vi "WPI_MotorControlClose.vi"(8 "error in (no error)":errorcluster, 11 "MotorControlDevRef":T1={"DeviceStatus"={"status"=FALSE, "code"=0, "source"=""}, "Type"=enum."PWM", "PWM"={"PWM Channel"=enum."PWM 1", "DeadBand"={"Name"="", "maxPositivePwm"=0, "minPositivePwm"=0, "centerPwm"=0, "maxNegativePwm"=0, "minNegativePwm"=0, "angularRange"=0}}, "CAN"={"Device Number"=0, "SetOutput VI Ref"=variant(enum8{"Percent VBus", "Current", "Speed", "Position", "Voltage"} enum."Percent VBus"), "GetOutput VI Ref"=variant(refnum<k1> refnum), "Enable VI Ref"=variant(dbl 12.0), "Disable VI Ref"=variant(enum8{"Percent VBus", "Speed", "Position", "Slave", "Unchanged / Invalid"} enum."Percent VBus"), "Data"=variant}, "Invert"=FALSE, "DIO PWM"={"PWM \"Enable\" Channel"=enum."Invalid", "DIOChannel"=enum."Invalid", "PWM Rate"=0.0}}) -> (0 "error out":errorcluster)   [LabVIEW 2017]
doc: "Closes the reference to the motor controller you specify. Use this VI to close each motor control reference that you open with the Open VI.\n\nThis software is licensed. Open the labview\\readme\\WPI Robotics Library Open Source License.txt file for more information."
uses:
  <vilib>/Rock Robotics/WPI/MotorControl/WPI_MotorControlDeviceRef.ctl
  <vilib>/Rock Robotics/WPI/MotorControl/WPI_MotorControlType.ctl
  <vilib>/Rock Robotics/SystemInterfaces/DIO/FPGA_DIOPWMChannel.ctl
  <vilib>/Rock Robotics/WPI/PWM/WPI_PWMDeadband.ctl
  <vilib>/Rock Robotics/SystemInterfaces/DIO/FPGA_DIOChannel.ctl
  <vilib>/Rock Robotics/WPI/PWM/WPI_PWMChannelCacheOp.ctl
  <instrlib>/DC Motor Controller/HAIOL/DC Motor Controller.lvclass
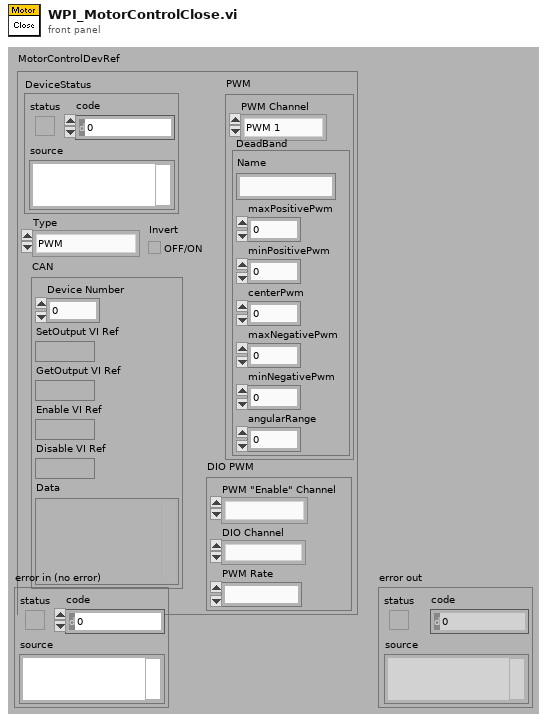
[diagram p1: front panel]
types:
  T1 = typedef "WPI_MotorControlDeviceRef.ctl" = cluster{"DeviceStatus":errorcluster, "Type":T2, "PWM":cluster{"PWM Channel":T3, "DeadBand":T4}, "CAN":cluster{"Device Number":u8, "SetOutput VI Ref":variant, "GetOutput VI Ref":variant, "Enable VI Ref":variant, "Disable VI Ref":variant, "Data":variant}, "Invert":bool, "DIO PWM":cluster{"PWM \"Enable\" Channel":T3, "DIOChannel":T5, "PWM Rate":dbl}}
  T2 = typedef "WPI_MotorControlType.ctl" = enum16{"PWM", "CAN", "DIO PWM"}
  T3 = typedef "FPGA_DIOPWMChannel.ctl" = enum8{"PWM 0", "PWM 1", "PWM 2", "PWM 3", "PWM 4", "PWM 5", "PWM 6", "PWM 7", "PWM 8", "PWM 9", "PWM MXP 0", "PWM MXP 1", "PWM MXP 2", "PWM MXP 3", "PWM MXP 4", "PWM MXP 5", "PWM MXP 6", "PWM MXP 7", "PWM MXP 8", "PWM MXP 9", "Invalid"}
  T4 = typedef "WPI_PWMDeadband.ctl" = cluster{"Name":string, "maxPositivePwm":i32, "minPositivePwm":i32, "centerPwm":i32, "maxNegativePwm":i32, "minNegativePwm":i32, "angularRange":u16}
  T5 = typedef "FPGA_DIOChannel.ctl" = enum8{"DIO 0", "DIO 1", "DIO 2", "DIO 3", "DIO 4", "DIO 5", "DIO 6", "DIO 7", "DIO 8", "DIO 9", "DIO MXP 0", "DIO MXP 1", "DIO MXP 2", "DIO MXP 3", "DIO MXP 4", "DIO MXP 5", "DIO MXP 6", "DIO MXP 7", "DIO MXP 8", "DIO MXP 9", "DIO MXP 10", "DIO MXP 11", "DIO MXP 12", "DIO MXP 13", "DIO MXP 14", "DIO MXP 15", "SPI Port CS1", "SPI Port CS2", "SPI Port CS3", "SPI Port MISO", "SPI Port MOSI", "Invalid"}
  T6 = typedef "WPI_PWMChannelCacheOp.ctl" = enum16{"Acquire", "Release", "Status"}
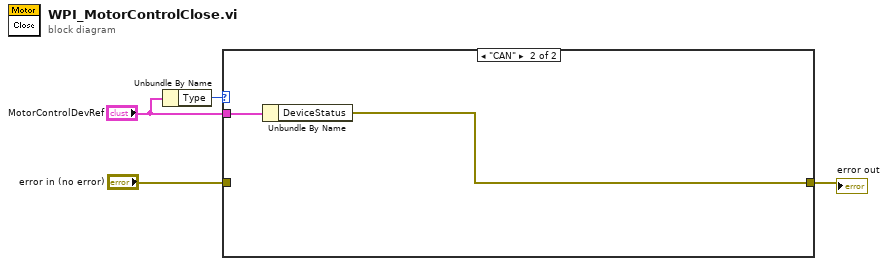
[diagram p0: block diagram]
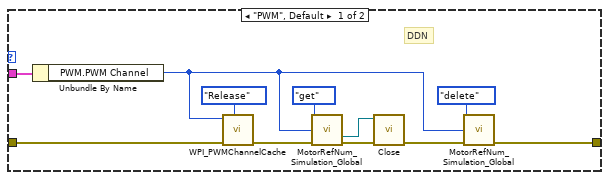
[diagram p2: hidden frame]
diagram:
  n1 = Unbundle By Name("MotorControlDevRef") -> ("Type"=w1:T2)
  n2 = case shown="\"CAN\"" w1 {
    tunnel: "error in (no error)" -> [w7 _]
    tunnel: [w6 w16] -> w3
    tunnel: "MotorControlDevRef" -> [w15 w17]
    frame "PWM", Default {
      # "DDN"
      n3 = Unbundle By Name(w15) -> ("PWM.PWM Channel"=w8:T3)
      n4 = call <vilib>:"WPI_PWMChannelCache.vi"("Operation"=WPI_PWMChannelCacheOp."Release", "error in (no error)"=w7, "PWMChannel"=w8) -> ("error out"=w12:errorcluster)  [unwired: 2 in, 6 out]
      n5 = call <vilib>:"MotorRefNum_Simulation_Global.vi"("menu"=enum16{"set", "get", "delete"}."get", "PWM Channel"=w8, "error in (no error)"=w12) -> ("DC Motor Controller Get"=w5:refnum<class "DC Motor Controller.lvclass">, "error out"=w11:errorcluster)  [unwired: 11 in]
      n6 = call-dynamic "Close.vi"("error in (no error)"=w11, "DC Motor Controller in"=w5) -> ("error out"=w9:errorcluster)  [unwired: 9 in]
      n7 = call <vilib>:"MotorRefNum_Simulation_Global.vi"("menu"=enum16{"set", "get", "delete"}."delete", "PWM Channel"=w8, "error in (no error)"=w9) -> ("error out"=w6:errorcluster)  [unwired: 11 in, 1 out]
    }
    frame "CAN" {
      n8 = Unbundle By Name(w17) -> ("DeviceStatus"=w16:errorcluster)
    }
  }
  "error out" <- w3
